vi "DVR.number_acq.Write.vi"(8 "error in":errorcluster, 10 "# acq":u16, 11 "DVR in":T1) -> (0 "error out":errorcluster)   [LabVIEW 2020]
uses:
  _controls/data.ctl
  camera/camera.lvclass
  _controls/data.ref.ctl
  <vilib>/vision/Image Controls.llb/IMAQ Image.ctl
  _controls/state.ctl
  _controls/data.vars.ctl
  _controls/save_options.ctl
  _controls/flip.ctl
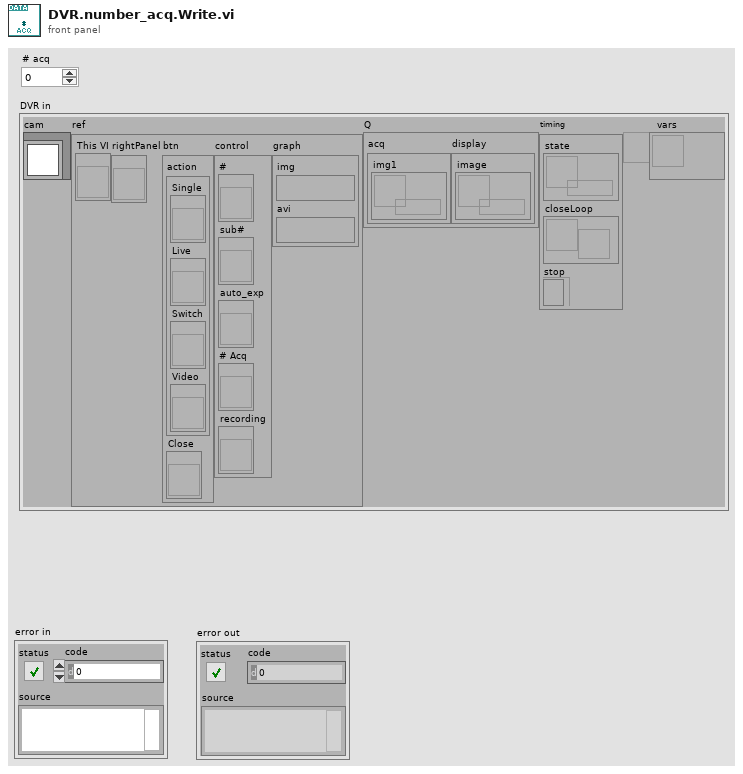
[diagram p1: front panel]
types:
  T1 = typedef "data.ctl" = cluster{"cam":refnum<class "camera.lvclass">, "ref":T2, "Q":cluster{"acq":cluster{"img1":refnum<queue>}, "display":cluster{"image":refnum<queue>}}, "timing":cluster{"state":refnum<queue>, "closeLoop":refnum<notifier>, "stop":refnum<k4>}, "vars":refnum<data-value>}
  T2 = typedef "data.ref.ctl" = cluster{"This VI":refnum<vi>, "rightPanel":refnum<vi>, "btn":cluster{"action":cluster{"Single":refnum<vi>, "Live":refnum<vi>, "Switch":refnum<vi>, "Video":refnum<vi>}, "Close":refnum<vi>}, "control":cluster{"#":refnum<vi>, "sub#":refnum<vi>, "auto_exp":refnum<vi>, "# Acq":refnum<vi>, "recording":refnum<vi>}, "graph":cluster{"img":T3, "avi":T3}}
  T3 = typedef "IMAQ Image.ctl" = refnum<image>
  T4 = typedef "data.vars.ctl" = cluster{"save":cluster{"base_folder":cluster{"Folder":path, "tif":bool, "jpg":bool}, "module":string, "#":u32, "sub#":u8, "save.op":T5, "same?":bool, "Shift":enum16{"Single", "Leapfrog"}, "jpg?":bool, "flip":T6}, "acq":cluster{"# Acq":u16, "rotate":bool, "FPS":dbl, "Test Mode":bool}, "calib.manual":cluster{"BG":cluster{"Image":u16[][], "enabled?":bool}, "FF":cluster{"Image":u16[][], "enabled?":bool}}}
  T5 = typedef "save_options.ctl" = enum16{"Light", "Full"}
  T6 = typedef "flip.ctl" = cluster{"x":bool, "y":bool}
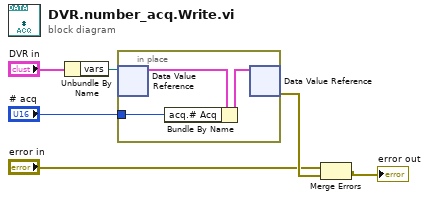
[diagram p0: block diagram]
diagram:
  n1 = Unbundle By Name("DVR in") -> ("vars"=w5:refnum<data-value>)
  n2 = in-place {
    in-place-border: "# acq" -> [w7]
    n3 = in-place-dvr #1(w5) -> (w9:T4)  [unwired: 1 out]
    n4 = Bundle By Name(cluster=w9, "acq.# Acq"=w7) -> (w8:T4)
    n5 = in-place-dvr #1(w8) -> (w6:errorcluster)  [unwired: 1 out]
  }
  n6 = Merge Errors("error in", w6) -> (→"error out":errorcluster)
